vi "ContextHelp_SendMessageToPopUp.vi"(1 "PopUpMessage":variant, 5 "error in (no error)":errorcluster) -> (19 "error out":errorcluster)   [LabVIEW 2016]
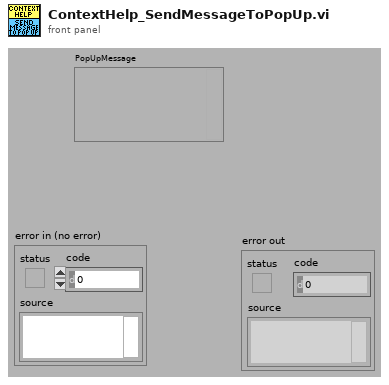
[diagram p1: front panel]
types:
  T1 = enum16{"SetPopUpEventTask", "GetStatus", "SetOpenState", "SetDialogCaller"}
  T2 = typedef "ContextHelp_EventType.ctl" = refnum<user-event>
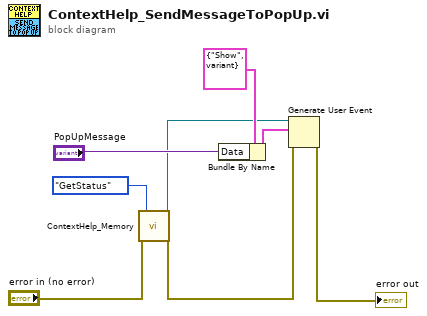
[diagram p0: block diagram]
diagram:
  n1 = call <resource>:"ContextHelp_Memory.vi"("error in (no error)"="error in (no error)", "Actio(GetStatus)n"=T1."GetStatus") -> ("PopUpTaskEventOut"=w4:T2, "error out"=w2:errorcluster)  [unwired: 2 in, 14 out]
  n2 = Bundle By Name(cluster=cluster{"Command":string, "Data":variant} {"Command"="Show", "Data"=variant} ("event data"), "Data"="PopUpMessage") -> (w8:cluster{"Command":string, "Data":variant})
  n3 = Generate User Event(user event=w4, event data cluster=w8, error in=w2) -> (error out=→"error out":errorcluster)  [unwired: 1 in, 1 out]
